vi "DSF.Engine.Execution.Builder.Parse.vi"(6 "Data Type Buffers in":T1, 8 "error in (no error)":errorcluster, 9 "Transfer ID":i32, 10 "Plugin ID":i32, 11 "Builder in":refnum<class "DSF.Engine.Execution.Builder.lvclass">) -> (0 "error out":errorcluster, 3 "Builder out":refnum<class "DSF.Engine.Execution.Builder.lvclass">, 4 "Data Type Buffers out":T1)   [LabVIEW 2016, in "DSF.Engine.lvlib" / "DSF.Engine.Execution.Builder.lvclass"]
uses:
  DSF.Engine.Execution.Builder.lvclass
  DSF.Engine.Execution.Builder.Type Buffers.ctl
  DSF.Engine.Execution.Builder.lvclass/DSF.Engine.Execution.Builder.ctl
  Cache/DSF.Engine.Memory.Cache.Framework.lvclass/DSF.Engine.Memory.Cache.Framework.ctl
  Cache/DSF.Engine.Memory.Cache.Plugin.lvclass/DSF.Engine.Memory.Cache.Plugin.ctl
  Cache/DSF.Engine.Memory.Cache.Transfer.lvclass/DSF.Engine.Memory.Cache.Transfer.ctl
  Submodules/Memory Manager/Source/Classes/Pointer/Memory.Pointer.lvclass/Memory.Pointer.ctl
  Pointer/DSF.Engine.Memory.Pointer.VS Channels.lvclass/DSF.Engine.Memory.Pointer.VS Channels.ctl
  Buffer/DSF.Engine.Memory.Buffer.Read.vi
  Buffer/DSF.Engine.Memory.Buffer.Read.1D.Bool.vi
  Buffer/DSF.Engine.Memory.Buffer.Read.1D.SGL.vi
  Buffer/DSF.Engine.Memory.Buffer.Read.1D.DBL.vi
  Buffer/DSF.Engine.Memory.Buffer.Read.1D.I8.vi
  Buffer/DSF.Engine.Memory.Buffer.Read.1D.I16.vi
  Buffer/DSF.Engine.Memory.Buffer.Read.1D.I32.vi
  Buffer/DSF.Engine.Memory.Buffer.Read.1D.I64.vi
  Buffer/DSF.Engine.Memory.Buffer.Read.1D.U8.vi
  Buffer/DSF.Engine.Memory.Buffer.Read.1D.U16.vi
  Buffer/DSF.Engine.Memory.Buffer.Read.1D.U32.vi
  Buffer/DSF.Engine.Memory.Buffer.Read.1D.U64.vi
  Cache/DSF.Engine.Memory.Cache.Framework.Get Plugin Caches.vi
  Cache/DSF.Engine.Memory.Cache.Plugin.Get Transfer Caches.vi
  Pointer/DSF.Engine.Memory.Pointer.VS Channels.Get Channel Count.vi
  Submodules/Memory Manager/Source/Classes/Pointer/Methods/Memory.Pointer.Write.vi
  Submodules/Memory Manager/Source/Classes/Pointer/Methods/Memory.Pointer.Write.Safe.1D.DBL.vi
  Submodules/Memory Manager/Source/Classes/Pointer/Methods/Memory.Pointer.Read.vi
  Submodules/Memory Manager/Source/Classes/Pointer/Methods/Memory.Pointer.Read.Safe.1D.Bool.vi
  Submodules/Memory Manager/Source/Classes/Pointer/Methods/Memory.Pointer.Read.Safe.1D.SGL.vi
  Submodules/Memory Manager/Source/Classes/Pointer/Methods/Memory.Pointer.Read.Safe.1D.DBL.vi
  Submodules/Memory Manager/Source/Classes/Pointer/Methods/Memory.Pointer.Read.Safe.1D.I8.vi
  Submodules/Memory Manager/Source/Classes/Pointer/Methods/Memory.Pointer.Read.Safe.1D.I16.vi
  Submodules/Memory Manager/Source/Classes/Pointer/Methods/Memory.Pointer.Read.Safe.1D.I32.vi
  Submodules/Memory Manager/Source/Classes/Pointer/Methods/Memory.Pointer.Read.Safe.1D.I64.vi
  Submodules/Memory Manager/Source/Classes/Pointer/Methods/Memory.Pointer.Read.Safe.1D.U8.vi
  Submodules/Memory Manager/Source/Classes/Pointer/Methods/Memory.Pointer.Read.Safe.1D.U16.vi
  Submodules/Memory Manager/Source/Classes/Pointer/Methods/Memory.Pointer.Read.Safe.1D.U32.vi
  Submodules/Memory Manager/Source/Classes/Pointer/Methods/Memory.Pointer.Read.Safe.1D.U64.vi
  Submodules/Memory Manager/Source/Classes/Pointer/Methods/Memory.Pointer.Write.Unsafe.1D.DBL.vi
  Submodules/Memory Manager/Source/Classes/Pointer/Methods/Memory.Pointer.Parameter Check.Null Pointer.vi
  Submodules/Memory Manager/Source/Classes/Pointer/Methods/Memory.Pointer.Parameter Check.Subset.Power of 2.vi
  Submodules/Memory Manager/Source/Classes/Pointer/Methods/Memory.Pointer.Read.Unsafe.1D.Bool.vi
  Submodules/Memory Manager/Source/Classes/Pointer/Methods/Memory.Pointer.Read.Unsafe.1D.SGL.vi
  Submodules/Memory Manager/Source/Classes/Pointer/Methods/Memory.Pointer.Read.Unsafe.1D.DBL.vi
  Submodules/Memory Manager/Source/Classes/Pointer/Methods/Memory.Pointer.Read.Unsafe.1D.I8.vi
  Submodules/Memory Manager/Source/Classes/Pointer/Methods/Memory.Pointer.Read.Unsafe.1D.I16.vi
  Submodules/Memory Manager/Source/Classes/Pointer/Methods/Memory.Pointer.Read.Unsafe.1D.I32.vi
  Submodules/Memory Manager/Source/Classes/Pointer/Methods/Memory.Pointer.Read.Unsafe.1D.I64.vi
  Submodules/Memory Manager/Source/Classes/Pointer/Methods/Memory.Pointer.Read.Unsafe.1D.U8.vi
  Submodules/Memory Manager/Source/Classes/Pointer/Methods/Memory.Pointer.Read.Unsafe.1D.U16.vi
  Submodules/Memory Manager/Source/Classes/Pointer/Methods/Memory.Pointer.Read.Unsafe.1D.U32.vi
  Submodules/Memory Manager/Source/Classes/Pointer/Methods/Memory.Pointer.Read.Unsafe.1D.U64.vi
  Submodules/Memory Manager/Source/Classes/Pointer/Accessors/Get Address.vi
  Submodules/Memory Manager/Source/Classes/Pointer/Methods/Memory.Pointer.Errors.vi
  Submodules/Memory Manager/Source/Classes/Pointer/Methods/Memory.Pointer.Errors.Null Pointer.vi
  Submodules/Memory Manager/Source/Classes/Pointer/Methods/Memory.Pointer.Errors.Out of Bounds.vi
  Submodules/Memory Manager/Source/Classes/Pointer/Accessors/Get Size.vi
  Submodules/Memory Manager/Source/VIs/Memory.Count to Size.Power of 2.vi
  Submodules/Memory Manager/Source/Classes/Pointer/Methods/Memory.Pointer.Errors.Create Error.vi
  Submodules/Memory Manager/Source/Submodules/SEH/Source/VIs/Static Error Handling.Source Buffer.Write.String.vi
  Submodules/Memory Manager/Source/Classes/Pointer/Methods/Memory.Pointer.Errors.Write Pointer Size.vi
  Submodules/Memory Manager/Source/Submodules/SEH/Source/VIs/Static Error Handling.Source Buffer.Write.Numeric.Scalar.Base10.vi
  Submodules/Memory Manager/Source/Submodules/SEH/Source/VIs/Static Error Handling.Source Buffer.Write.Numeric.Scalar.Base10 (U64).vi
  Submodules/Memory Manager/Source/Submodules/SEH/Source/VIs/Static Error Handling.Error Cluster Constant.vi
  Submodules/Memory Manager/Source/Submodules/SEH/Source/VIs/Static Error Handling.Error Cluster Constant (256B).vi
  Submodules/Memory Manager/Source/Submodules/SEH/Source/VIs/Static Error Handling.Parameters.Status.Set.vi
  Submodules/Memory Manager/Source/Submodules/SEH/Source/VIs/Static Error Handling.Parameters.Code.Set.vi
  Submodules/Memory Manager/Source/Submodules/SEH/Source/VIs/Static Error Handling.Parameters.VI Source.Set.vi
  Submodules/Memory Manager/Source/Constants/Memory.Constants.vi
  Submodules/Memory Manager/Source/Constants/Memory.Constants.Library Name.vi
  Submodules/Memory Manager/Source/Classes/Pointer/Methods/Memory.Pointer.Errors.Get Info.vi
  Buffer/DSF.Engine.Memory.Buffer.lvclass
  C:/Git/Sourcetree/DSF/Source/Submodules/Memory Manager/Source/Classes/Pointer/Memory.Pointer.lvclass
  Pointer/DSF.Engine.Memory.Pointer.VS Channels.lvclass
  Cache/DSF.Engine.Memory.Cache.Framework.lvclass
  Cache/DSF.Engine.Memory.Cache.Plugin.lvclass
  Cache/DSF.Engine.Memory.Cache.Transfer.lvclass
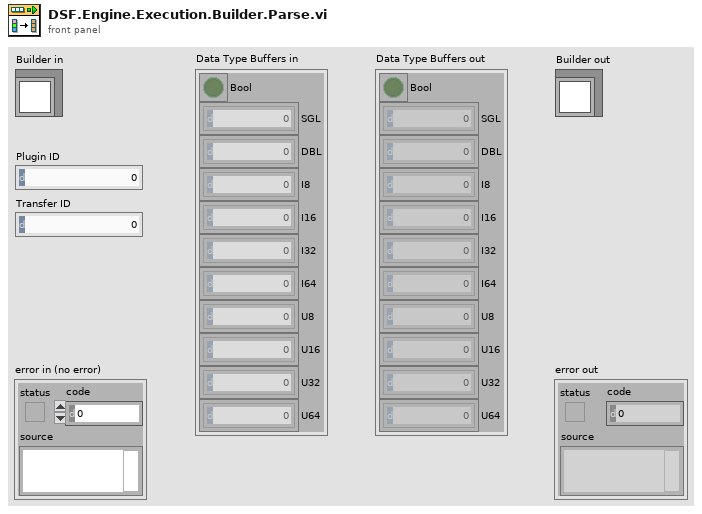
[diagram p1: front panel]
types:
  T1 = typedef "DSF.Engine.lvlib/DSF.Engine.Execution.Builder.lvclass/DSF.Engine.Execution.Builder.Type Buffers.ctl" = cluster{"Bool":bool[], "SGL":sgl[], "DBL":dbl[], "I8":i8[], "I16":i16[], "I32":i32[], "I64":i64[], "U8":u8[], "U16":u16[], "U32":u32[], "U64":u64[]}
  T2 = typedef "DSF.Engine.lvlib/DSF.Engine.Buffer Channel Configuration.ctl" = cluster{"data type":T3, "offset":u64, "count":u64, "index":u64}
  T3 = typedef "DSF.Shared.lvlib/DSF.Shared.Data Type.ctl" = enum8{"Bool", "SGL", "DBL", "I8", "I16", "I32", "I64", "U8", "U16", "U32", "U64"}
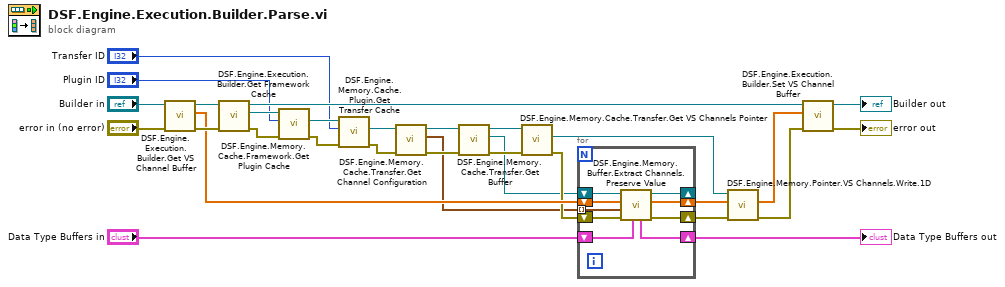
[diagram p0: block diagram]
diagram:
  n1 = call "DSF.Engine.Execution.Builder.Get VS Channel Buffer.vi"("error in (no error)"="error in (no error)", "Builder in"="Builder in") -> ("error out"=w25:errorcluster, "VS Channel Buffer"=w17:dbl[], "Builder out"=w26:refnum<class "DSF.Engine.Execution.Builder.lvclass">)  [unwired: 7 in]
  n2 = call "DSF.Engine.Execution.Builder.Get Framework Cache.vi"("error in (no error)"=w25, "Builder in"=w26) -> ("error out"=w27:errorcluster, "Framework Cache"=w30:refnum<class "DSF.Engine.Memory.Cache.Framework.lvclass">, "Builder out"=w24:refnum<class "DSF.Engine.Execution.Builder.lvclass">)  [unwired: 7 in]
  n3 = call "DSF.Engine.Memory.Cache.Framework.Get Plugin Cache.vi"("error in (no error)"=w27, "Plugin ID"="Plugin ID", "Framework Cache in"=w30) -> ("error out"=w28:errorcluster, "Plugin Cache"=w29:refnum<class "DSF.Engine.Memory.Cache.Plugin.lvclass">)  [unwired: 6 in, 1 out]
  n4 = call "DSF.Engine.Memory.Cache.Plugin.Get Transfer Cache.vi"("error in (no error)"=w28, "Transfer ID"="Transfer ID", "Plugin Cache in"=w29) -> ("error out"=w8:errorcluster, "Transfer Cache"=w5:refnum<class "DSF.Engine.Memory.Cache.Transfer.lvclass">)  [unwired: 6 in, 1 out]
  n5 = call "DSF.Engine.Memory.Cache.Transfer.Get Channel Configuration.vi"("error in (no error)"=w8, "Transfer Cache in"=w5) -> ("error out"=w7:errorcluster, "Channel Configuration"=w2:T2[], "Transfer Cache out"=w4:refnum<class "DSF.Engine.Memory.Cache.Transfer.lvclass">)  [unwired: 7 in]
  n6 = call "DSF.Engine.Memory.Cache.Transfer.Get Buffer.vi"("error in (no error)"=w7, "Transfer Cache in"=w4) -> ("error out"=w6:errorcluster, "Buffer"=w1:refnum<class "DSF.Engine.Memory.Buffer.lvclass">, "Transfer Cache out"=w3:refnum<class "DSF.Engine.Memory.Cache.Transfer.lvclass">)  [unwired: 7 in]
  n7 = call "DSF.Engine.Memory.Cache.Transfer.Get VS Channels Pointer.vi"("error in (no error)"=w6, "Transfer Cache in"=w3) -> ("error out"=w14:errorcluster, "VS Channels Pointer"=w11:refnum<class "DSF.Engine.Memory.Pointer.VS Channels.lvclass">)  [unwired: 7 in, 1 out]
  n8 = for {
    tunnel: w2 -> [w34] mode=indexing
    shift-right: [w37] -> w15
    shift-left: w17 -> [w38]
    shift-right: [w36] -> w16
    shift-left: w14 -> [w39]
    shift-right: [w32] -> w9
    shift-left: "Data Type Buffers in" -> [w33]
    shift-right: [w31] -> _
    shift-left: w1 -> [w35]
    n9 = call "DSF.Engine.Memory.Buffer.Extract Channels.Preserve Value.vi"("Data Type Buffers in"=w33, "error in (no error)"=w39, "Channel Configuration"=w34, "VS Channels Array in"=w38, "Buffer in"=w35) -> ("error out"=w36:errorcluster, "VS Channels Array out"=w37:dbl[], "Buffer out"=w31:refnum<class "DSF.Engine.Memory.Buffer.lvclass">, "Data Type Buffers out"=w32:T1)  [unwired: 3 in]
  }
  "Data Type Buffers out" <- w9
  n10 = call "DSF.Engine.Memory.Pointer.VS Channels.Write.1D.vi"("error in (no error)"=w16, "Channels Array in"=w15, "VS Channels Pointer in"=w11) -> ("error out"=w13:errorcluster, "Channels Array out"=w12:dbl[])  [unwired: 5 in, 2 out]
  n11 = call "DSF.Engine.Execution.Builder.Set VS Channel Buffer.vi"("error in (no error)"=w13, "VS Channel Buffer"=w12, "Builder in"=w24) -> ("error out"=→"error out":errorcluster, "Builder out"=→"Builder out":refnum<class "DSF.Engine.Execution.Builder.lvclass">)  [unwired: 7 in]
